vi "Execute Value Update Policy.vi"(8 "error in (no error)":errorcluster, 9 "Publish Time":timestamp, 10 "New Topic Value":variant, 11 "OneShotSubscription In":refnum<class "OneShotSubscription.lvclass">) -> (0 "error out":errorcluster, 3 "OneShotSubscription Out":refnum<class "OneShotSubscription.lvclass">)   [LabVIEW 2017, in "SubscriptionPolicy.lvlib" / "OneShotSubscription.lvclass"]
uses:
  OneShotSubscription.lvclass
  C:/Git/mva-framework/Source/Framework/IMediator/ISubscriptionPolicy/ISubscriptionPolicy.lvclass
  IMediator/ISubscriptionPolicy/ISubscriptionPolicy.lvclass/ISubscriptionPolicy.ctl
  gpm_packages/@cs/transport/Source/ITransport/Transport Data.vi
  <vilib>/Utility/error.llb/Error Cluster From Error Code.vi
  <vilib>/ErrorRing/Error Ring.xnode
  gpm_packages/@cs/transport/Source/ITransport/ITransport.lvclass
  IMediator/ISubscriptionPolicy/ISubscriptionPolicy.lvclass
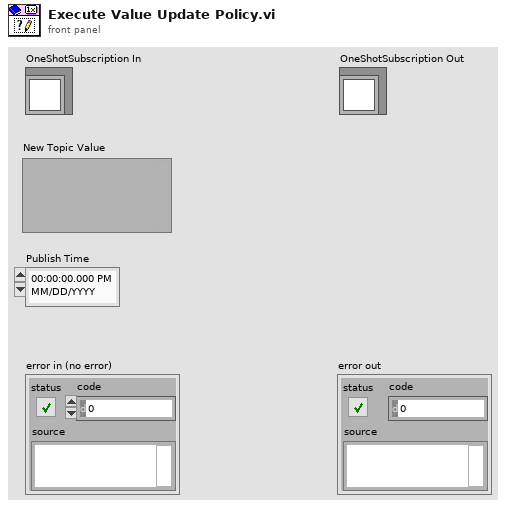
[diagram p1: front panel]
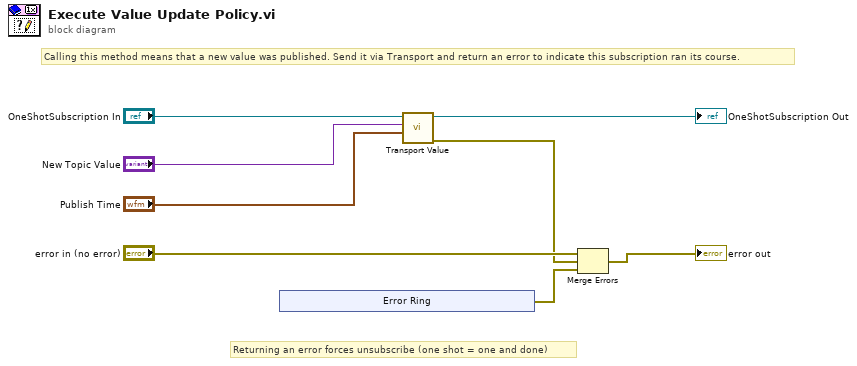
[diagram p0: block diagram]
diagram:
  # "Calling this method means that a new value was published. Send it via Transport and return an error to indicate this subscription ran its course."
  # "Returning an error forces unsubscribe (one shot = one and done)"
  n1 = xnode "Error Ring"() -> ("error out"=w6:errorcluster)
  n2 = call "Transport Value.vi"("Publish Time"="Publish Time", "Value"="New Topic Value", "ISubscriptionPolicy in"="OneShotSubscription In") -> ("error out"=w3:errorcluster, "ISubscriptionPolicy out"=→"OneShotSubscription Out":refnum<class "OneShotSubscription.lvclass">)  [unwired: 7 in]
  n3 = Merge Errors("error in (no error)", w3, w6) -> (→"error out":errorcluster)
